vi "Util.Cmprs.LZW.CU.BitStream__ogtk.vi"(6 "Bits":i32, 8 "error in (no error)":errorcluster, 9 "Chars in":u8[](array[numeric]) format="%.0b", 10 "Codes in":i16[](array[numeric]), 11 "PackUnpack":bool) -> (0 "error out":errorcluster, 1 "Codes out":i16[](array[numeric]), 2 "Chars out":u8[](array[numeric]) format="%.0x")   [LabVIEW 2018]
panel:
  out "Error":bool
  # "LZW.CU.BitStream.vi\n\nPacks or unpacks bit-packed LZW codes\".\n \n\nPlease visit http://www.OpenG.org to learn about the\nOpen Source LabVIEW software movement.\n\nNOTICE -- YOU MUST LEAVE THIS NOTICE IN PLACE.  PER THE TERMS OF THE LICENSE BELOW, YOU MAY SUBLICENSE THIS SOFTWARE \nIN ANY WAY THAT DOES NOT CONFLICT WITH THIS LICENSE.\n\n### BSD License (http://www.opensource.org/licenses/bsd-license.php) Begin ###\n \nCopyright (c) 2007, Bill Clench <bclench@yahoo.com>\n\nAll rights reserved.\n\nRedistribution and use in source and binary forms, with or without modification, are permitted provided that the following conditions are met:\n\n    * Redistributions of source code must retain the above copyright notice, this list of conditions and the following disclaimer.\n    * Redistributions in binary form must reproduce the above copyright notice, this list of conditions and the following disclaimer in the \n       documentation and/or other materials provided with the distribution.\n    * Neither the name of SciWare, James Kring, Inc., nor the names of its contributors may be used to endorse or promote products derived \n       from this software without specific prior written permission.\n\nTHIS SOFTWARE IS PROVIDED BY THE COPYRIGHT HOLDERS AND CONTRIBUTORS \"AS IS\" AND ANY EXPRESS OR IMPLIED WARRANTIES, \nINCLUDING, BUT NOT LIMITED TO, THE IMPLIED WARRANTIES OF MERCHANTABILITY AND FITNESS FOR A PARTICULAR PURPOSE ARE \nDISCLAIMED. IN NO EVENT SHALL THE COPYRIGHT OWNER OR CONTRIBUTORS BE LIABLE FOR ANY DIRECT, INDIRECT, INCIDENTAL,\n SPECIAL, EXEMPLARY, OR CONSEQUENTIAL DAMAGES (INCLUDING, BUT NOT LIMITED TO, PROCUREMENT OF SUBSTITUTE GOODS OR \nSERVICES; LOSS OF USE, DATA, OR PROFITS; OR BUSINESS INTERRUPTION) HOWEVER CAUSED AND ON ANY THEORY OF LIABILITY, \nWHETHER IN CONTRACT, STRICT LIABILITY, OR TORT (INCLUDING NEGLIGENCE OR OTHERWISE) ARISING IN ANY WAY OUT OF THE USE \nOF THIS SOFTWARE, EVEN IF ADVISED OF THE POSSIBILITY OF SUCH DAMAGE.\n\n### BSD License End ###"
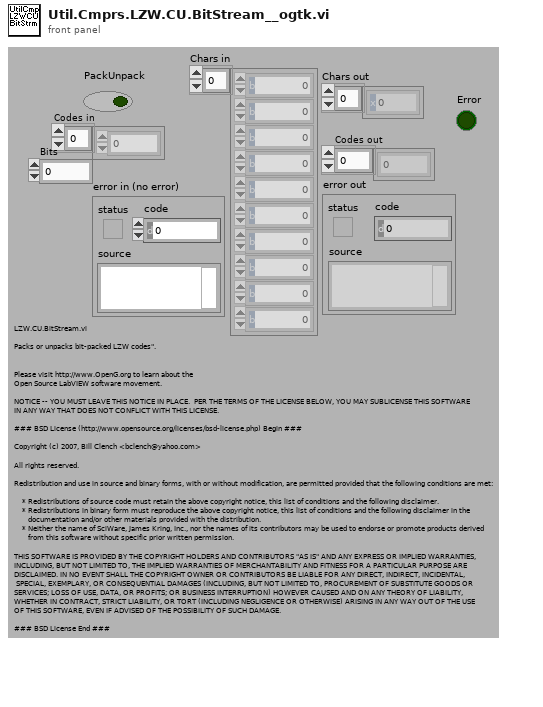
[diagram p1: front panel]
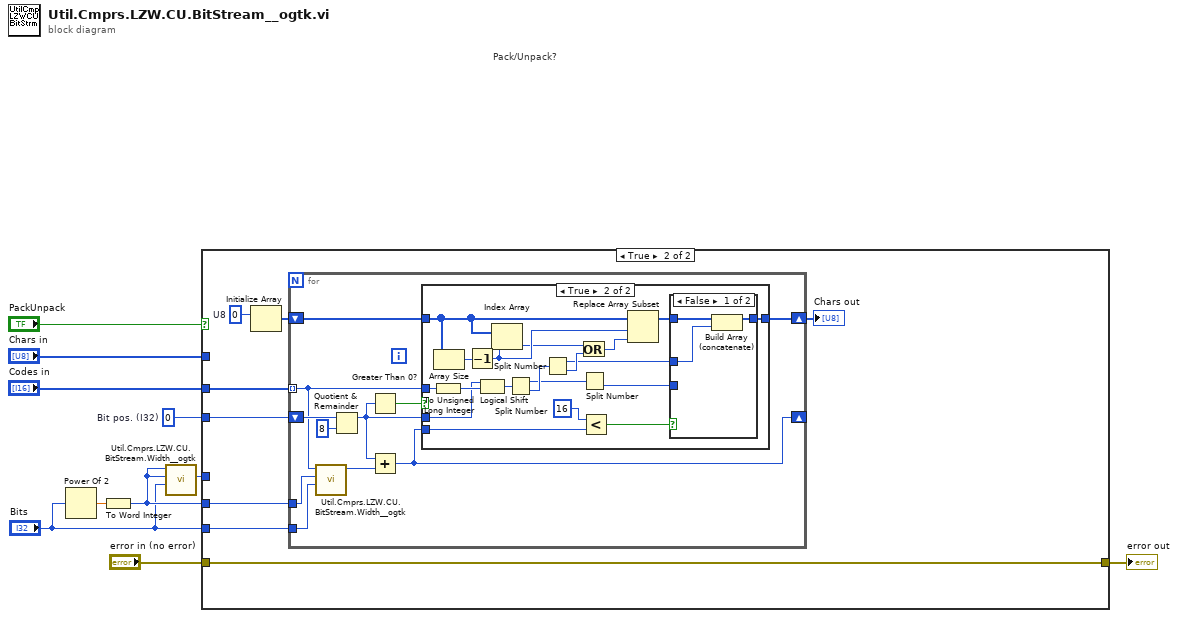
[diagram p0: block diagram]
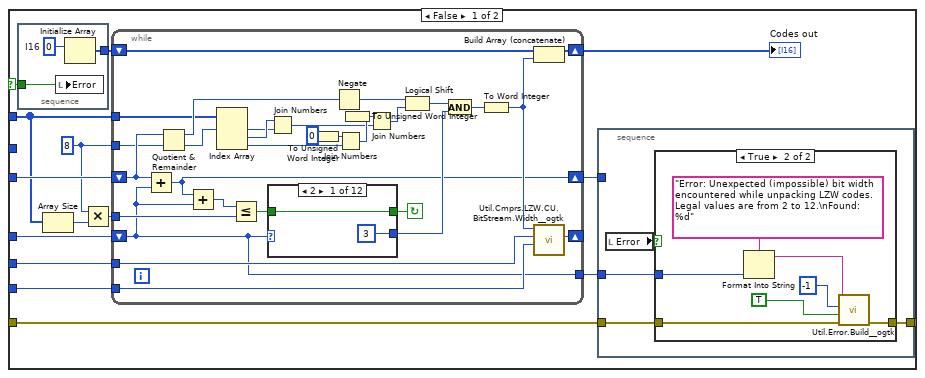
[diagram p2: hidden frame]
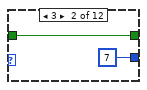
[diagram p4: hidden frame]
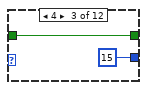
[diagram p5: hidden frame]
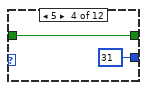
[diagram p6: hidden frame]
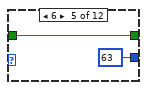
[diagram p7: hidden frame]
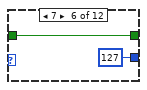
[diagram p8: hidden frame]
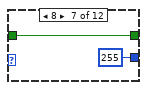
[diagram p9: hidden frame]
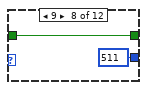
[diagram p10: hidden frame]
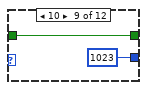
[diagram p11: hidden frame]
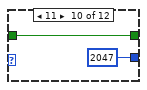
[diagram p12: hidden frame]
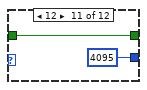
[diagram p13: hidden frame]
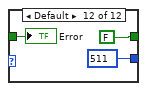
[diagram p14: hidden frame]
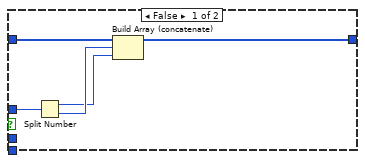
[diagram p15: hidden frame]
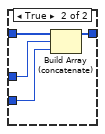
[diagram p16: hidden frame]
diagram:
  w7 = 0  # Bit pos. (I32)
  # "Pack/Unpack?"
  n1 = Power Of 2(x="Bits") -> (2^x=w5:dbl)
  n2 = To Word Integer(number=w5) -> (16bit integer=w4:i16)
  n3 = call <userlib>:"Util.Cmprs.LZW.CU.BitStream.Width__ogtk.vi"("ImageBits"="Bits", "Reset"=w4, "Code"=w4) -> ("Bit Width next"=w6:i32)  [unwired: 7 in, 1 out]
  n4 = case shown="True" "PackUnpack" {
    selector: "PackUnpack" -> [w16 _]
    tunnel: "Codes in" -> [_ w102]
    tunnel: "Chars in" -> [w23 _]
    tunnel: w7 -> [w25 w101]
    tunnel: w6 -> [w20 _]
    tunnel: "Bits" -> [w19 w98]
    tunnel: w4 -> [w18 w97]
    tunnel: "error in (no error)" -> [w14 w96]
    tunnel: [w12 w96] -> w1
    frame False {
      w17 = 8 ("x")
      n5 = stacked-sequence {
        tunnel: [w39] -> w24
        tunnel: w16 -> [w38]
        frame #0 {
          w40 = i16 0  # I16
          n6 = local write "Error"(w38) -> ()
          n7 = Initialize Array(w40) -> (w39:i16[])  [unwired: 1 in]
        }
      }
      n8 = Array Size(array=w23) -> (size(s)=w22:i32)
      n9 = Multiply(x=w17, y=w22) -> (x*y=w21:i32)
      n10 = while {
        tunnel: w23 -> [w58]
        shift-right: [w50] -> w11
        shift-left: w25 -> [w54]
        shift-right: [w49] -> _
        shift-left: w20 -> [w43]
        shift-right: [w55] -> w15
        shift-left: w24 -> [w56]
        tunnel: w21 -> [w52]
        tunnel: w19 -> [w48]
        tunnel: w18 -> [w47]
        tunnel: w17 -> [w46]
        tunnel: [w43] -> w13
        stop <- w44 continue-if-true
        n11 = Add(x=w54, y=w43) -> (x+y=w50:i32)
        n12 = Quotient & Remainder(x=w54, y=w46) -> (x-y*floor(x/y)=w59:i32, floor(x/y)=w57:i32)
        n13 = Add(x=w50, y=w43) -> (x+y=w53:i32)
        n14 = Index Array(array=w58, index #1=w57) -> (element #1=w60:u8, element #2=w62:u8, element #3=w61:u8)  [unwired: 2 in]
        n15 = Less Or Equal?(x=w53, y=w52) -> (x <= y?=w45:bool)
        n16 = Join Numbers(hi=w62, lo=w60) -> ((hi.lo)=w63:u16)
        n17 = case shown="2" w43 {
          tunnel: [u32 3 u32 7 u32 15 u32 31 u32 63 u32 127 u32 255 u32 511 u32 1023 u32 2047 u32 4095 u32 511] -> w66
          tunnel: w45 -> [w71 w73 w75 w77 w79 w81 w83 w85 w87 w89 w91 w93]
          tunnel: [w71 w73 w75 w77 w79 w81 w83 w85 w87 w89 w91 FALSE] -> w44
          frame 2 {
          }
          frame 3 {
          }
          frame 4 {
          }
          frame 5 {
          }
          frame 6 {
          }
          frame 7 {
          }
          frame 8 {
          }
          frame 9 {
          }
          frame 10 {
          }
          frame 11 {
          }
          frame 12 {
          }
          frame Default {
            "Error" <- w93
          }
        }
        n18 = To Unsigned Word Integer(number=0) -> (unsigned 16bit integer=w41:u16)
        n19 = Negate(x=w59) -> (-x=w67:i32)
        n20 = Join Numbers(hi=w41, lo=w61) -> ((hi.lo)=w64:u32)
        n21 = To Unsigned Word Integer(number=w64) -> (unsigned 16bit integer=w42:u16)
        n22 = Join Numbers(hi=w42, lo=w63) -> ((hi.lo)=w65:u32)
        n23 = Logical Shift(y=w67, x=w65) -> (x << y=w70:u32)
        n24 = And(x=w70, y=w66) -> (x .and. y?=w68:u32)
        n25 = To Word Integer(number=w68) -> (16bit integer=w51:i16)
        n26 = Build Array (concatenate)(w56, w51) -> (w55:i16[])
        n27 = call <userlib>:"Util.Cmprs.LZW.CU.BitStream.Width__ogtk.vi"("ImageBits"=w48, "Reset"=w47, "Code"=w51) -> ("Bit Width next"=w49:i32)  [unwired: 7 in, 1 out]
      }
      "Codes out" <- w15
      n28 = stacked-sequence {
        tunnel: w14 -> [w27]
        tunnel: w13 -> [w28]
        tunnel: [w26] -> w12
        tunnel: w11 -> [_]
        frame #0 {
          n29 = local read "Error"() -> (w29:bool)
          n30 = case shown="True" w29 {
            tunnel: w28 -> [_ w36]
            tunnel: w27 -> [w30 w35]
            tunnel: [w30 w34] -> w26
            frame False {
            }
            frame True {
              n31 = Format Into String(format string="Error: Unexpected (impossible) bit width encountered while unpacking LZW codes.  Legal values are from 2 to 12.\nFound: %d", w36) -> (resulting string=w33:string)  [unwired: 2 in, 1 out]
              n32 = call <userlib>:"Util.Error.Build__ogtk.vi"("error in (no error)"=w35, "Status"=TRUE, "code"=-1, "Source"=w33) -> ("error out"=w34:errorcluster)  [unwired: 7 in]
            }
          }
        }
      }
    }
    frame True {
      w100 = u8 0  # U8
      n33 = Initialize Array(w100) -> (w99:u8[])  [unwired: 1 in]
      n34 = for {
        tunnel: w102 -> [w107] mode=indexing
        shift-right: [w111] -> _
        shift-left: w101 -> [w114]
        shift-right: [w113] -> w103
        shift-left: w99 -> [w112]
        tunnel: w98 -> [w105]
        tunnel: w97 -> [w104]
        n35 = call <userlib>:"Util.Cmprs.LZW.CU.BitStream.Width__ogtk.vi"("ImageBits"=w105, "Reset"=w104, "Code"=w107) -> ("Bit Width"=w106:i32)  [unwired: 7 in, 1 out]
        n36 = Quotient & Remainder(x=w114, y=8) -> (x-y*floor(x/y)=w108:i32)  [unwired: 1 out]
        n37 = Greater Than 0?(x=w108) -> (x > 0?=w109:bool)
        n38 = Add(x=w108, y=w106) -> (x+y=w111:i32)
        n39 = case shown="True" w109 {
          tunnel: w112 -> [w119 w132]
          tunnel: w107 -> [w118 w138]
          tunnel: [w115 w126] -> w113
          tunnel: w108 -> [_ w123]
          tunnel: w111 -> [_ w121]
          frame False {
            n40 = Split Number(x=w118) -> (hi(x)=w116:u8, lo(x)=w117:u8)
            n41 = Build Array (concatenate)(w119, w117, w116) -> (w115:u8[])
          }
          frame True {
            n42 = To Unsigned Long Integer(number=w138) -> (unsigned 32bit integer=w137:u32)
            n43 = Array Size(array=w132) -> (size(s)=w134:i32)
            n44 = Decrement(x=w134) -> (x-1=w131:i32)
            n45 = Logical Shift(y=w123, x=w137) -> (x << y=w136:u32)
            n46 = Index Array(array=w132, index=w131) -> (element=w130:u8)
            n47 = Split Number(x=w136) -> (hi(x)=w125:u16, lo(x)=w135:u16)
            n48 = Split Number(x=w135) -> (hi(x)=w127:u8, lo(x)=w128:u8)
            n49 = Or(x=w130, y=w128) -> (x .or. y?=w129:u8)
            n50 = Split Number(x=w125) -> (lo(x)=w124:u8)  [unwired: 1 out]
            n51 = Less?(x=16, y=w121) -> (x < y?=w122:bool)
            n52 = Replace Array Subset(array=w132, new element=w129, index=w131) -> (w133:u8[])
            n53 = case shown="False" w122 {
              tunnel: w133 -> [w141 w145]
              tunnel: w127 -> [w140 w143]
              tunnel: [w139 w144] -> w126
              tunnel: w124 -> [_ w142]
              frame False {
                n54 = Build Array (concatenate)(w141, w140) -> (w139:u8[])
              }
              frame True {
                n55 = Build Array (concatenate)(w145, w143, w142) -> (w144:u8[])
              }
            }
          }
        }
      }
      "Chars out" <- w103
    }
  }
  "error out" <- w1
